vi "Var Tools Speed.vi"() -> ()   [LabVIEW 2015]
uses:
  <vilib>/Utility/Data Type/Type Definitions/Data Type.ctl
  <vilib>/Utility/VariantDataType/VariantType.lvlib
  <vilib>/Utility/Data Type/NI_Data Type.lvlib
panel:
  out "x/y":dbl format="%#_6p"
  out "Array":T1[](array[typedef])
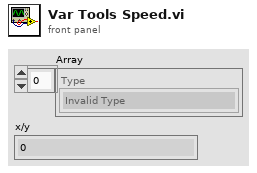
[diagram p1: front panel]
types:
  T1 = typedef "NI_Data Type.lvlib/Data Type.ctl" = enum8{"Invalid Type", "Void", "I8", "I16", "I32", "I64", "U8", "U16", "U32", "U64", "Single Float", "Double Float", "Extended Float", "Single Complex", "Double Complex", "Extended Complex", "Enum U8", "Enum U16", "Enum U32", "Enum U64", "Single Float With Unit", "Double Float With Unit", "Extended Float With Unit", "Single Complex with Unit", "Double Complex with Unit", "Extended Complex with Unit", "Boolean", "String", "Path", "Picture", "Tag", "Array", "Cluster", "Variant", "LV Variant", "Waveform", "Timestamp", "Digital Waveform", "Digital Data", "ExpressData", "Refnum", "External Data", "VI", "Poly VI", "LabVIEW Class Instance", "Fixed Point"}
  T2 = cluster{"enum":enum16{"dsdsf", "sdagads", "gsd", "gsgvdsg"}, "1":dbl, string}
  T3 = typedef "VariantType.lvlib/Type.ctl" = enum8{"Invalid Type", "Void", "I8", "I16", "I32", "I64", "U8", "U16", "U32", "U64", "Single Float", "Double Float", "Extended Float", "Single Complex", "Double Complex", "Extended Complex", "Enum U8", "Enum U16", "Enum U32", "Enum U64", "Single Float With Unit", "Double Float With Unit", "Extended Float With Unit", "Single Complex with Unit", "Double Complex with Unit", "Extended Complex with Unit", "Boolean", "String", "Path", "Picture", "Tag", "Array", "Cluster", "Variant", "LV Variant", "Waveform", "Timestamp", "Digital Waveform", "Digital Data", "ExpressData", "Refnum", "External Data", "VI", "Poly VI", "LabVIEW Class Instance", "Fixed Point"}
  T4 = typedef "NI_Data Type.lvlib/Type Definition Info.ctl" = cluster{"Name":string, "Timestamp":u32}
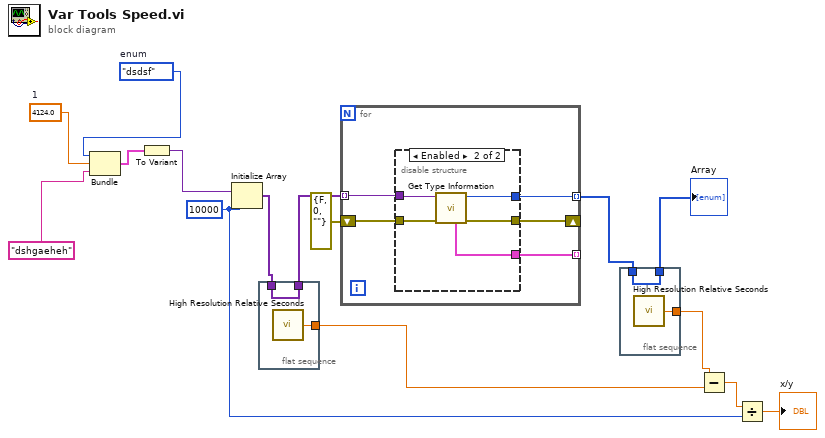
[diagram p0: block diagram]
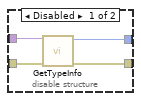
[diagram p2: hidden frame]
diagram:
  w3 = 4124.0  # 1
  w4 = enum16{"dsdsf", "sdagads", "gsd", "gsgvdsg"}."dsdsf"  # enum
  w7 = 10000 ("dimension size")
  n1 = Bundle("enum"=w4, "1"=w3, "dshgaeheh") -> (w1:T2)  [unwired: 1 in]
  n2 = To Variant(anything=w1) -> (Variant=w15:variant)
  n3 = Initialize Array(w15, w7) -> (w13:variant[])
  n4 = flat-sequence {
    tunnel: w13 -> [w17]
    tunnel: [w17] -> w12
    tunnel: [w16] -> w9
    frame #0 {
      n5 = call <vilib>:"High Resolution Relative Seconds.vi"() -> ("relative seconds"=w16:dbl)
    }
  }
  n6 = for {
    tunnel: w12 -> [w22] mode=indexing
    tunnel: [w21] -> w11 mode=indexing
    shift-right: [w20] -> _
    shift-left: errorcluster {"status"=FALSE, "code"=0, "source"=""} ("error out") -> [w19]
    tunnel: [w18] -> _ mode=indexing
    n7 = disable-structure shown="Enabled" {
      disable-tunnel: w22 -> [w26 w31]
      disable-tunnel: [w25 w30] -> w21
      disable-tunnel: [w24 w28] -> w20
      disable-tunnel: w19 -> [w23 w29]
      disable-tunnel: [_ w27] -> w18
      frame Disabled {
        n8 = call <vilib>:"GetTypeInfo.vi"("error in (no error)"=w23, "Variant"=w26) -> ("error out"=w24:errorcluster, "Type Enum"=w25:T3)  [unwired: 5 in, 3 out]
      }
      frame Enabled {
        n9 = call <vilib>:"Get Type Information.vi"("error in (no error)"=w29, "Variant"=w31) -> ("error out"=w28:errorcluster, "Type"=w30:T1, "Type Definition Info"=w27:T4)  [unwired: 5 in, 2 out]
      }
    }
  }
  n10 = flat-sequence {
    tunnel: w11 -> [w33]
    tunnel: [w33] -> w5
    tunnel: [w32] -> w10
    frame #0 {
      n11 = call <vilib>:"High Resolution Relative Seconds.vi"() -> ("relative seconds"=w32:dbl)
    }
  }
  n12 = Subtract(x=w10, y=w9) -> (x-y=w8:dbl)
  n13 = Divide(x=w8, y=w7) -> (x/y=→"x/y":dbl)
  "Array" <- w5
